vi "ex_openTDMForReading.vi"(6 "Plugin info":T2, 7 "storage_format":T1, 8 "error in (no error)":errorcluster, 9 "read info  in":T3, 10 "Reset":bool, 11 "file path in":path) -> (0 "error out":errorcluster, 1 "description":string, 3 "read info  out":T3)   [LabVIEW 2020]
uses:
  <vilib>/Platform/express/TDMExpress.llb/ex_readInfoTDM.ctl
  <vilib>/Platform/express/TDMExpress.llb/ex_readChannelInfo.ctl
  <vilib>/express/express shared/ExFile.llb/ex_TdmData.ctl
  <vilib>/express/express shared/ExFile.llb/ex_TdmProperty.ctl
  <vilib>/express/express shared/ex_EditUserDefinedProperties/usiDataType.ctl
  <vilib>/express/express shared/ExFile.llb/ex_PluginInfo.ctl
  <vilib>/express/express shared/ExFile.llb/ex_FileFormatSelector.ctl
  <vilib>/Platform/storage/lvStorage.llb/_openFunction.ctl
  <vilib>/Platform/storage/lvStorage.llb/_wf_attributes.ctl
  <vilib>/Platform/storage/Storage.llb/__loadPropTime.vi
  <vilib>/Platform/storage/Storage.llb/__loadPropString.vi
  <vilib>/Platform/storage/Storage.llb/__loadPropRefList.vi
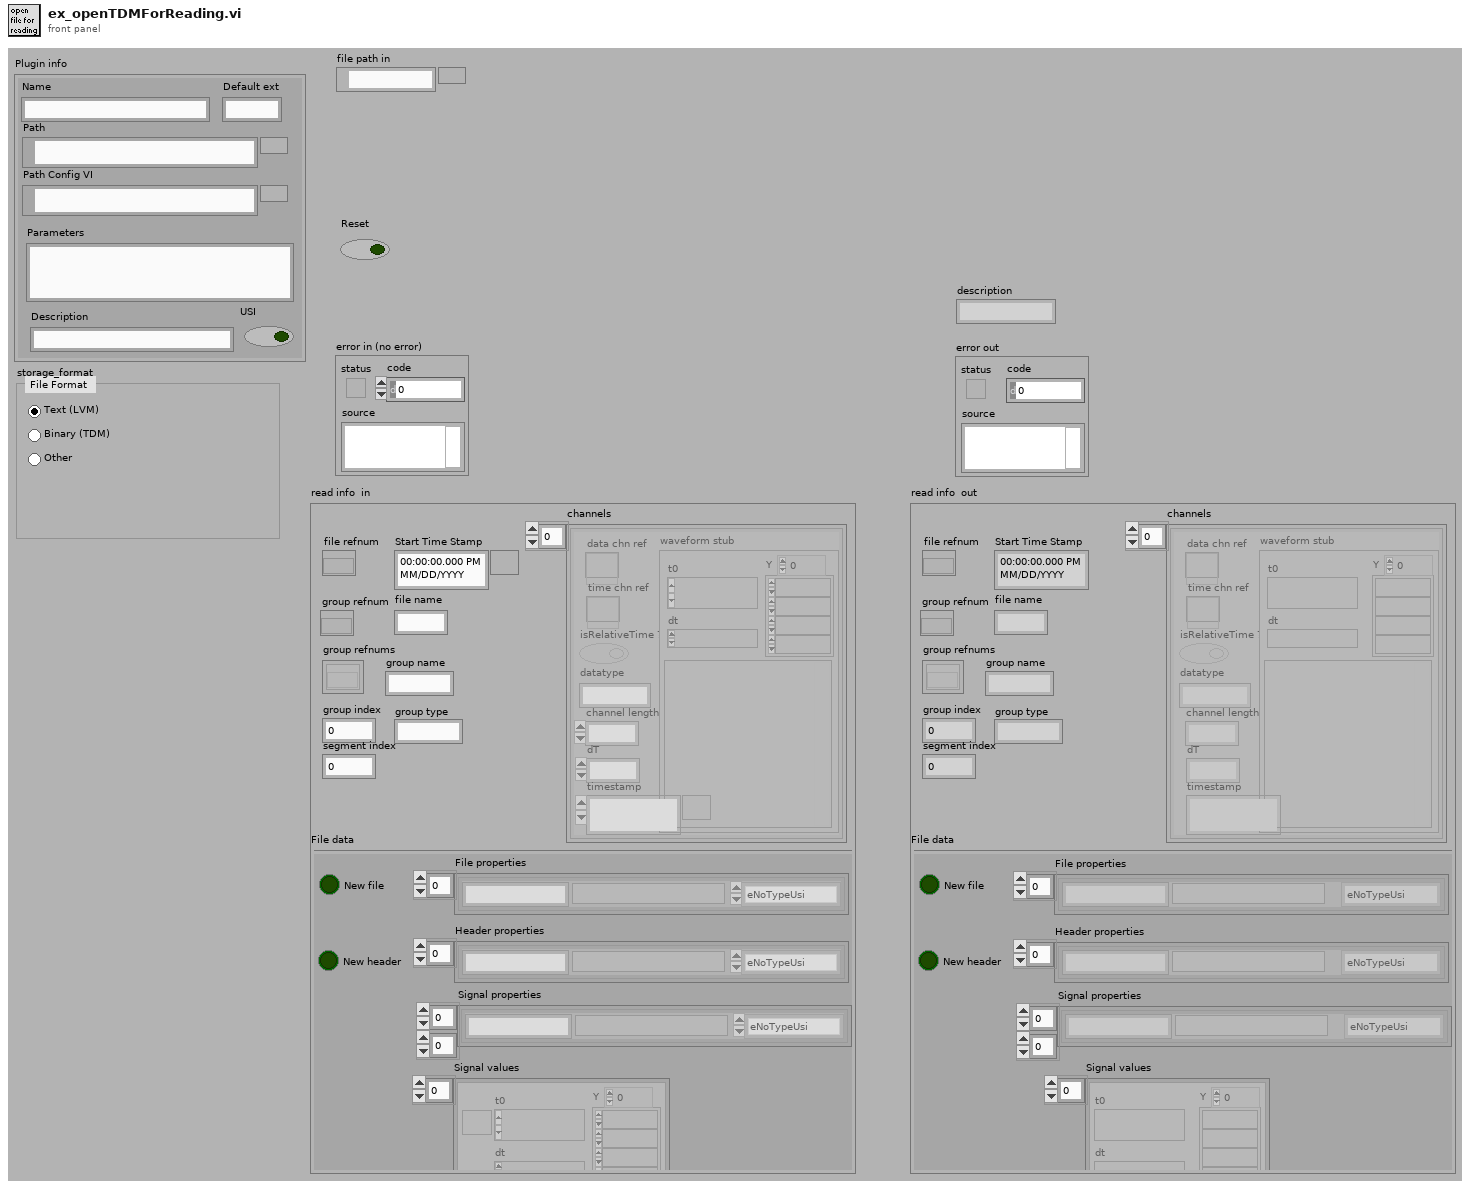
[diagram p1: front panel]
types:
  T1 = typedef "ex_FileFormatSelector.ctl" = enum32{"lvm", "tdm", "other"}
  T2 = typedef "ex_PluginInfo.ctl" = cluster{"Name":string, "Path":path, "Default ext":string, "Parameters":string, "Path Config VI":path, "Description":string, "USI":bool}
  T3 = typedef "ex_readInfoTDM.ctl" = cluster{"file refnum":refnum<k20>, "group refnum":refnum<k20>, "group name":string, "group type":string, "Start Time Stamp":timestamp, "group index":u32, "group refnums":refnum<k20>[], "file name":string, "segment index":u32, "channels":T4[], "File data":T5}
  T4 = typedef "ex_readChannelInfo.ctl" = cluster{"data chn ref":refnum<k20>, "time chn ref":refnum<k20>, "isRelativeTime ?":bool, "channel length":u32, "dT":dbl, "waveform stub":waveform(dbl), "datatype":string, "timestamp":timestamp}
  T5 = typedef "ex_TdmData.ctl" = cluster{"New file":bool, "New header":bool, "File properties":T6[], "Header properties":T6[], "Signal properties":T6[][], "Signal values":waveform(dbl)[]}
  T6 = typedef "ex_TdmProperty.ctl" = cluster{"Name":string, "Type":T7, "Value":variant}
  T7 = typedef "usiDataType.ctl" = enum16{"eNoTypeUsi", "eInt8Usi", "eInt16Usi", "eInt32Usi", "eInt64Usi", "eUInt8Usi", "eUInt16Usi", "eUInt32Usi", "eUInt64Usi", "eFloat32Usi", "eFloat64Usi", "- 0", "- 1", "- 2", "- 3", "- 4", "- 5", "- 6", "- 7", "- 8", "- 9", "eString8Usi", "eString16Usi", "eStringUsi", "eEnumUsi", "- 10", "- 11", "- 12", "- 13", "- 14", "eTimeUsi", "- 15", "- 16", "- 17", "- 18", "- 19", "- 20", "- 21", "- 22", "- 23", "eInstanceUsi", "eStoreUsi"}
  T8 = typedef "_wf_attributes.ctl" = enum16{"t0", "dt", "X_Name", "X_Unit", "x0", "abs/rel", "nPoints", "file_timestamp", "xcolumns"}
  T9 = typedef "_openFunction.ctl" = enum16{"open", "open or create", "create or replace", "create", "open (read only)"}
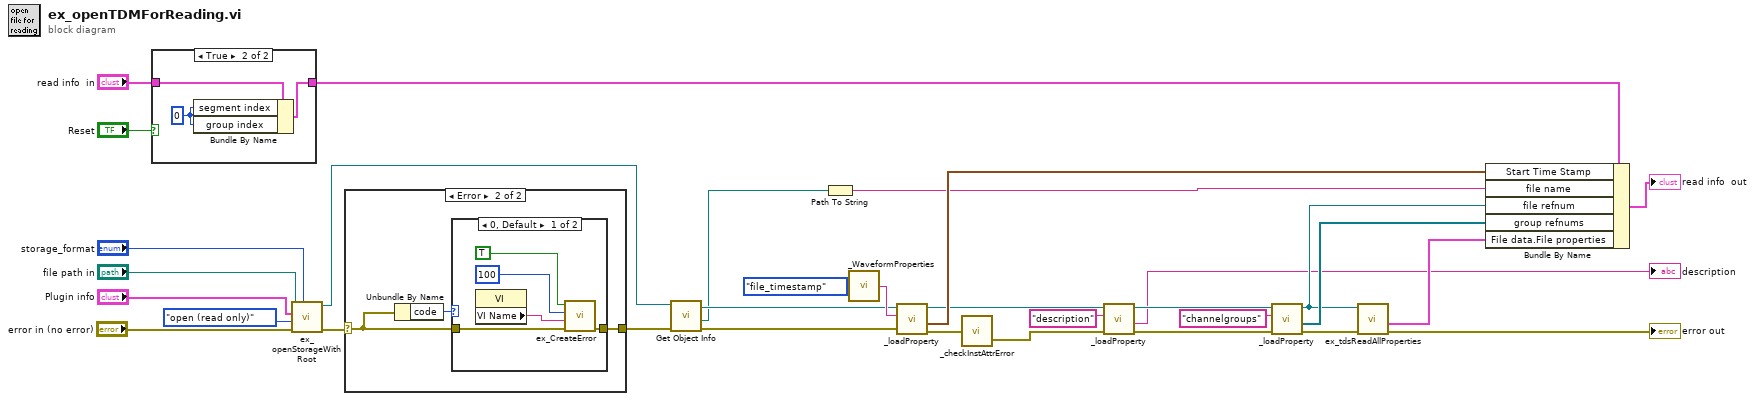
[diagram p0: block diagram]
diagram:
  n1 = case shown="True" "Reset" {
    tunnel: "read info  in" -> [w33 w35]
    tunnel: [w33 w34] -> w13
    frame False {
    }
    frame True {
      w36 = u32 0 ("group index")
      n2 = Bundle By Name(cluster=w35, "segment index"=w36, "group index"=w36) -> (w34:T3)
    }
  }
  n3 = call <vilib>:"ex_openStorageWithRoot.vi"("storage_format"="storage_format", "error in (no error)"="error in (no error)", "Overwrite Options"=_openFunction."open (read only)", "Plugin info"="Plugin info", "Storage Location"="file path in") -> ("error out"=w1:errorcluster, "Data Object"=w8:refnum<k20>)  [unwired: 5 out]
  n4 = case shown="Error" w1 {
    selector: w1 -> [w37 w39]
    tunnel: [w37 w40] -> w2
    frame No Error {
    }
    frame Error {
      n5 = Unbundle By Name(w39) -> ("code"=w38:i32)
      n6 = case shown="0, Default" w38 {
        tunnel: [w45 w46] -> w40
        tunnel: w39 -> [w41 w46]
        frame 0, Default {
          n7 = property class="VI"() -> ("VI Name"=w42:string)  [unwired: 2 in, 2 out]
          n8 = call <vilib>:"ex_CreateError.vi"("error in (no error)"=w41, "source"=w42, "code"=100, "error?"=TRUE) -> ("error out"=w45:errorcluster)  [unwired: 7 out]
        }
        frame 43 {
        }
      }
    }
  }
  n9 = call <vilib>:"Get Object Info.vi"("error in (no error)"=w2, "storage refnum"=w8) -> ("error out"=w10:errorcluster, "storage location"=w4:path, "storage refnum out"=w9:refnum<k20>)  [unwired: 7 out]
  n10 = Path To String(path=w4) -> (string=w3:string)
  n11 = call <vilib>:"_WaveformProperties.vi"("Property"=_wf_attributes."file_timestamp") -> ("Name"=w21:string)
  n12 = call-poly <vilib>:"_loadProperty.vi"("error in (no error)"=w10, "Property name"=w21, "storage refnum"=w9) -> ("error out"=w20:errorcluster, "Value"=w24:timestamp, "dup storage refnum"=w23:refnum<k20>)  [unwired: 6 out]
  n13 = call <vilib>:"_checkInstAttrError.vi"("error in (no error)"=w20) -> ("error out"=w19:errorcluster)  [unwired: 1 out]
  n14 = call-poly <vilib>:"_loadProperty.vi"("error in (no error)"=w19, "Property name"="description" ("property name"), "storage refnum"=w23) -> ("error out"=w29:errorcluster, "Value"=→"description":string, "dup storage refnum"=w28:refnum<k20>)  [unwired: 6 out]
  n15 = call-poly <vilib>:"_loadProperty.vi"("error in (no error)"=w29, "Property name"="channelgroups" ("Object type"), "storage refnum"=w28) -> ("error out"=w12:errorcluster, "Value"=w32:refnum<k20>[], "dup storage refnum"=w15:refnum<k20>)  [unwired: 6 out]
  n16 = call <vilib>:"ex_tdsReadAllProperties.vi"("error in (no error)"=w12, "Data Object in"=w15) -> ("error out"=→"error out":errorcluster, "Properties Out"=w14:T6[])  [unwired: 4 out]
  n17 = Bundle By Name(cluster=w13, "Start Time Stamp"=w24, "file name"=w3, "file refnum"=w15, "group refnums"=w32, "File data.File properties"=w14) -> (→"read info  out":T3)
